vi "CountersVisualization.vi"(0 "Counters Monitor Array IN":T1(array[cluster]), 1 "SenderMail":string, 3 "ConnectionDSN":string, 4 "Password":string, 5 "Recipients":string, 6 "ArrayAlarmIN":bool[](array[boolean]), 7 "LineName":string, 9 "PLC Connection Array":T3(array[cluster]) {"PLC Type" items=["Keyence", "Allen Bradley", "Mitsubishi", "Panasonic", "Siemens"]}, 11 "OnlineStations":T2(array[cluster]), 13 "EmailsEnabled":string) -> (14 "Counters Monitor Array OUT":T1(array[cluster]), 19 "ArrayAlarmOUT":bool[](array[boolean]))   [LabVIEW 2017]
panel:
  in  "Tab Control":enum32{"Parameters", "Components", "Machines"}(tab)
  # "Online Monitor"
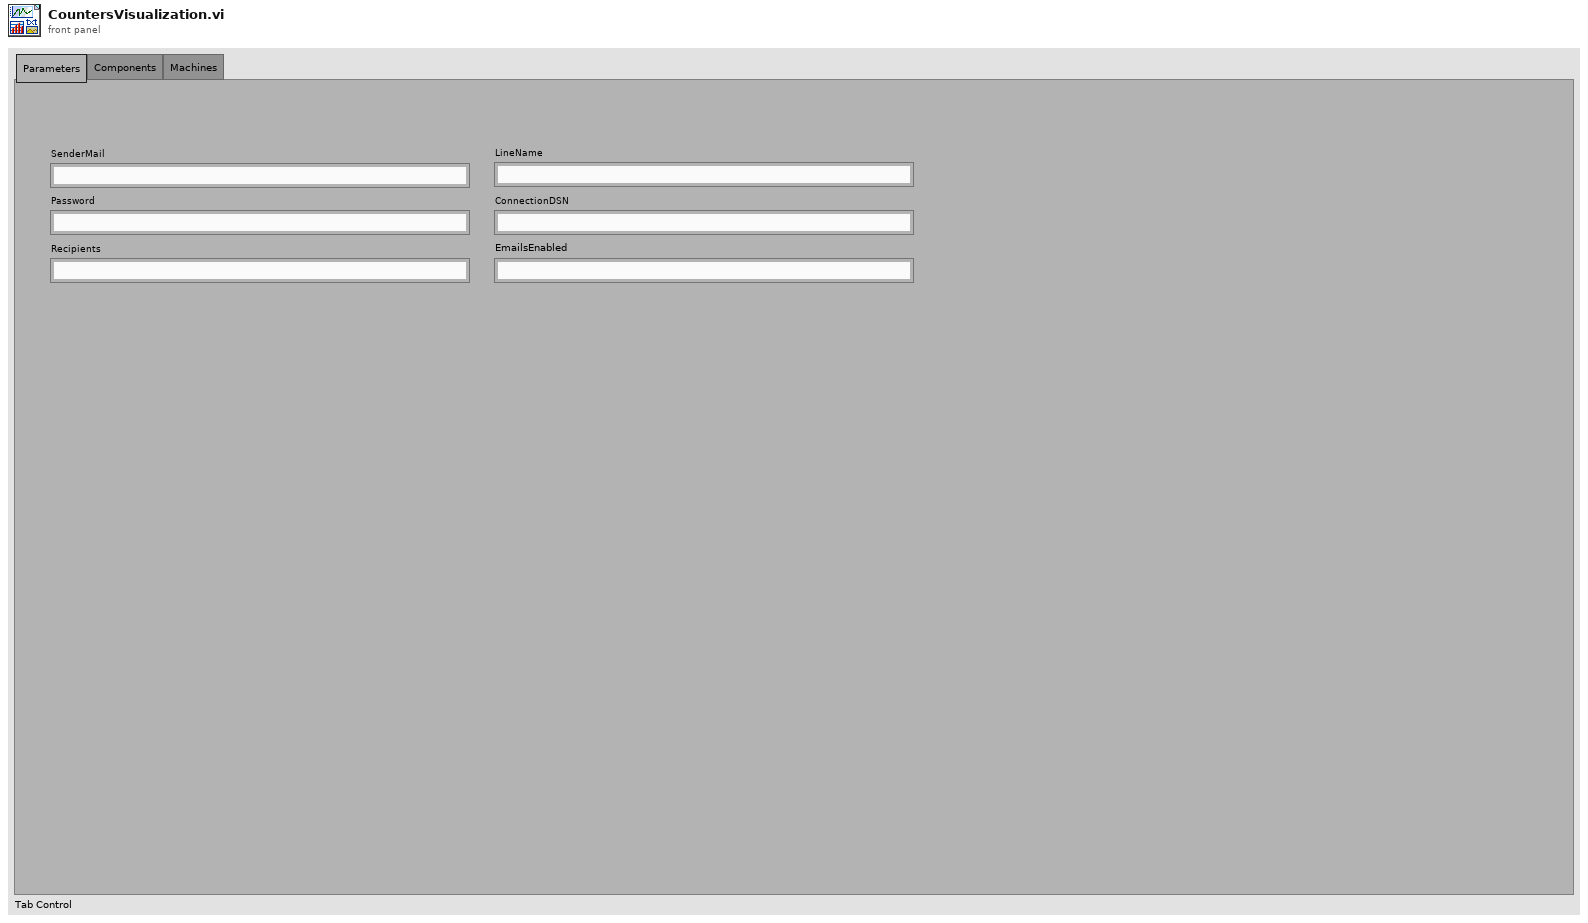
[diagram p1: front panel]
types:
  T1 = cluster{"MachineName":string, "ComponentName":string, "StoppageAlarmCounter":i32, "CurrentCount":i32, "StatusColorBox":u32, "ToolCribPartNumber":string}[]
  T2 = cluster{"Connection":bool, "MachineName":string}[]
  T3 = cluster{"MachineName":string, "PLC Address":string, "PLC Type":u16, "MemoryNumber1":string, "MemoryNumber2":string, "MemoryNumber3":string}[]
  T4 = enum8{"Enabled", "Disabled", "Disabled and Grayed Out"}
  T5 = cluster{"MachineName":string, "ComponentName":string, "StoppageAlarmCounter":i32, "CurrentCount":i32, "StatusColorBox":u32, "ToolCribPartNumber":string}
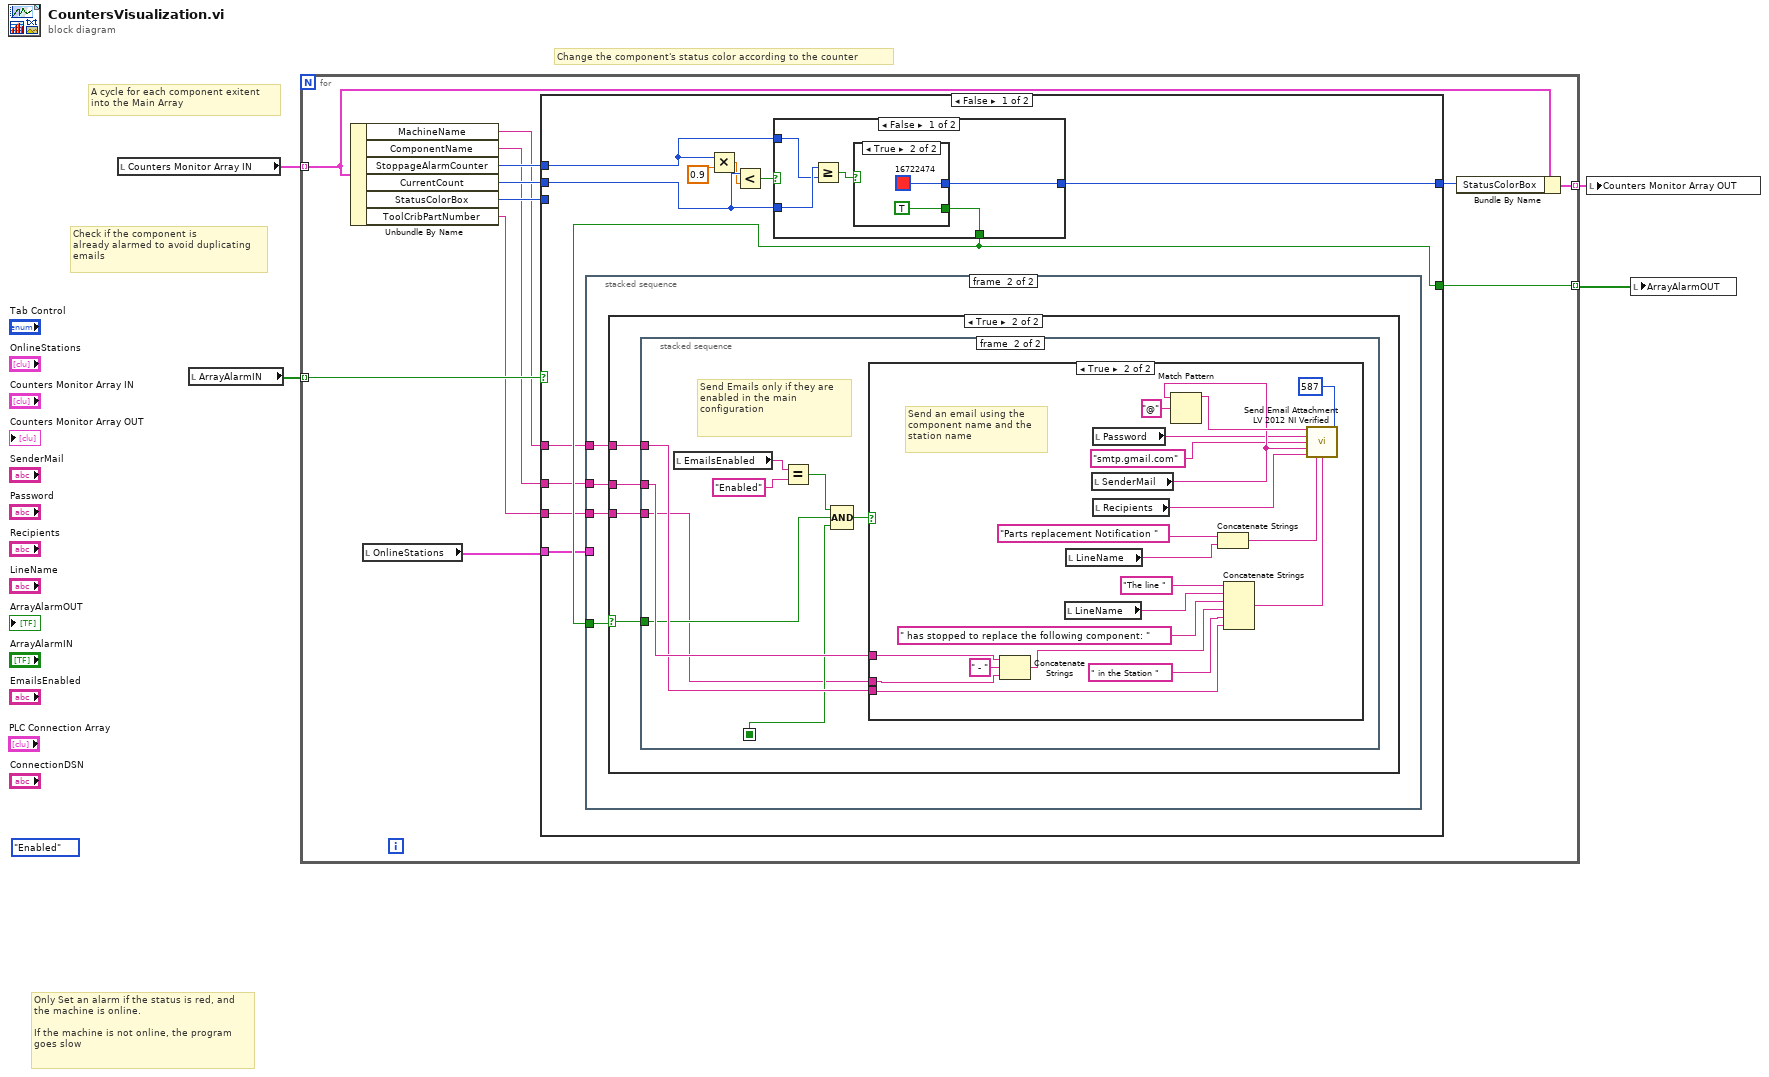
[diagram p0: block diagram]
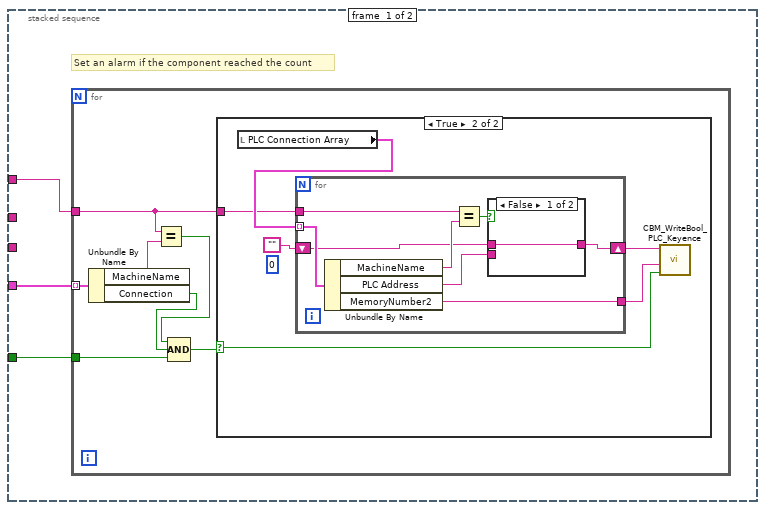
[diagram p2: hidden frame]
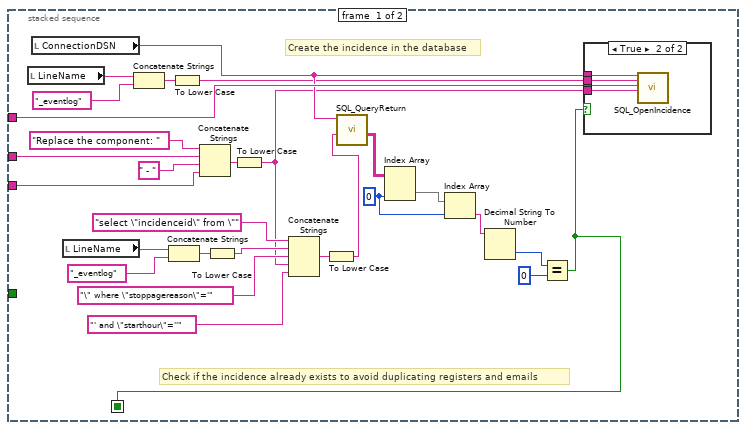
[diagram p6: hidden frame]
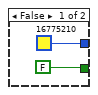
[diagram p9: hidden frame]
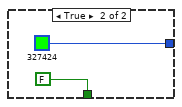
[diagram p10: hidden frame]
diagram:
  (unwired) T4."Enabled" ("Disabled")
  # "Only Set an alarm if the status is red, and\nthe machine is online.\n\nIf the machine is not online, the program \ngoes slow"
  # "Change the component's status color according to the counter"
  # "Check if the component is \nalready alarmed to avoid duplicating\nemails"
  # "A cycle for each component exitent\ninto the Main Array"
  n1 = local read "Counters Monitor Array IN"() -> (w4:T1)
  n2 = local read "ArrayAlarmIN"() -> (w2:bool[])
  n3 = for {
    tunnel: w4 -> [w16] mode=indexing
    tunnel: [w14] -> w3 mode=indexing
    tunnel: w2 -> [w12] mode=indexing
    tunnel: [w11] -> w1 mode=indexing
    n4 = Unbundle By Name(w16) -> ("MachineName"=w8:string, "ComponentName"=w6:string, "StoppageAlarmCounter"=w13:i32, "CurrentCount"=w10:i32, "StatusColorBox"=w9:u32, "ToolCribPartNumber"=w5:string)
    n5 = local read "OnlineStations"() -> (w7:T2)
    n6 = case shown="False" w12 {
      selector: w12 -> [_ w135]
      tunnel: [w25 w134] -> w15
      tunnel: w10 -> [w24 _]
      tunnel: w13 -> [w22 _]
      tunnel: [w21 w135] -> w11
      tunnel: w9 -> [_ w134]
      tunnel: w8 -> [w20 _]
      tunnel: w7 -> [w19 _]
      tunnel: w6 -> [w18 _]
      tunnel: w5 -> [w17 _]
      frame False {
        n7 = Multiply(x=w22, y=0.9) -> (x*y=w23:dbl)
        n8 = Less?(x=w24, y=w23) -> (x < y?=w26:bool)
        n9 = case shown="False" w26 {
          tunnel: [w124 u32 327424] -> w25
          tunnel: w24 -> [w127 _]
          tunnel: w22 -> [w126 _]
          tunnel: [w123 FALSE] -> w21
          frame False {
            n10 = Greater Or Equal?(x=w127, y=w126) -> (x >= y?=w125:bool)
            n11 = case shown="True" w125 {
              tunnel: [u32 16775210 u32 16722474] -> w124
              tunnel: [FALSE TRUE] -> w123
              frame False {
              }
              frame True {
              }
            }
          }
          frame True {
          }
        }
        n12 = stacked-sequence {
          tunnel: w21 -> [w30 w54]
          tunnel: w20 -> [w29 w57]
          tunnel: w19 -> [w28 _]
          tunnel: w18 -> [_ w56]
          tunnel: w17 -> [_ w55]
          frame #0 {
            # "Set an alarm if the component reached the count"
            n13 = for {
              tunnel: w30 -> [w31]
              tunnel: w29 -> [w36]
              tunnel: w28 -> [w37] mode=indexing
              n14 = Unbundle By Name(w37) -> ("MachineName"=w35:string, "Connection"=w32:bool)
              n15 = Equal?(x=w36, y=w35) -> (x = y?=w33:bool)
              n16 = Compound Arithmetic op=AND(w33, w32, w31) -> (w34:bool)
              n17 = case shown="True" w34 {
                selector: w34 -> [_ w41]
                tunnel: w36 -> [_ w42]
                frame False {
                }
                frame True {
                  (unwired) 0
                  n18 = local read "PLC Connection Array"() -> (w43:T3)
                  n19 = for {
                    tunnel: w43 -> [w51] mode=indexing
                    tunnel: w42 -> [w49]
                    shift-right: [w46] -> w40
                    shift-left: "" -> [w45]
                    tunnel: [w44] -> w38
                    n20 = Unbundle By Name(w51) -> ("MachineName"=w50:string, "PLC Address"=w47:string, "MemoryNumber2"=w44:string)
                    n21 = Equal?(x=w49, y=w50) -> (x = y?=w48:bool)
                    n22 = case shown="False" w48 {
                      tunnel: w47 -> [_ w53]
                      tunnel: [w52 w53] -> w46
                      tunnel: w45 -> [w52 _]
                      frame False {
                      }
                      frame True {
                      }
                    }
                  }
                  n23 = call "CBM_WriteBool_PLC_Keyence.vi"("Set?"=w41, "MemoryNumber"=w38, "PLC_IP"=w40) -> ()  [unwired: 8 in, 1 out]
                }
              }
            }
          }
          frame #1 {
            n24 = case shown="True" w54 {
              selector: w54 -> [_ w58]
              tunnel: w57 -> [_ w61]
              tunnel: w56 -> [_ w60]
              tunnel: w55 -> [_ w59]
              frame False {
              }
              frame True {
                n25 = stacked-sequence {
                  seq-local: [w62 _] -> [_ w96]
                  tunnel: w61 -> [w87 w101]
                  tunnel: w60 -> [w85 w102]
                  tunnel: w59 -> [w83 w94]
                  tunnel: w58 -> [_ w97]
                  frame #0 {
                    w70 = 0 ("disabled index (col)")
                    # "Check if the incidence already exists to avoid duplicating registers and emails"
                    # "Create the incidence in the database"
                    n26 = local read "LineName"() -> (w89:string)
                    n27 = local read "ConnectionDSN"() -> (w81:string)
                    n28 = local read "LineName"() -> (w76:string)
                    n29 = Concatenate Strings(w89, "_eventlog") -> (w82:string)
                    n30 = Concatenate Strings(w76, "_eventlog") -> (w78:string)
                    n31 = To Lower Case(string=w82) -> (all lower case string=w80:string)
                    n32 = Concatenate Strings("Replace the component: " ("Subject:"), w85, " - " ("Subject:"), w83) -> (w64:string)
                    n33 = To Lower Case(string=w78) -> (all lower case string=w75:string)
                    n34 = To Lower Case(string=w64) -> (all lower case string=w63:string)
                    n35 = Concatenate Strings("select \"incidenceid\" from \"", w75, "\" where \"stoppagereason\"='", w63, "' and \"starthour\"=''") -> (w69:string)
                    n36 = To Lower Case(string=w69) -> (all lower case string=w68:string)
                    n37 = call "SQL_QueryReturn.vi"("SQL query"=w68, "ConnectionDSN"=w81) -> ("data"=w72:string[][])  [unwired: 9 in]
                    n38 = Index Array(array=w72, index (col)=w70) -> (element=w71:string[])  [unwired: 1 in]
                    n39 = Index Array(array=w71, index=w70) -> (element=w67:string)
                    n40 = Decimal String To Number(string=w67) -> (number=w66:i32)  [unwired: 2 in, 1 out]
                    n41 = Equal?(x=w66, y=0) -> (x = y?=w62:bool)
                    n42 = case shown="True" w62 {
                      tunnel: w81 -> [_ w93]
                      tunnel: w87 -> [_ w92]
                      tunnel: w63 -> [_ w91]
                      tunnel: w80 -> [_ w90]
                      frame False {
                      }
                      frame True {
                        n43 = call "SQL_OpenIncidence.vi"("ConnectionDSN"=w93, "TableName"=w90, "MachineName"=w92, "StoppageReason"=w91) -> ()  [unwired: 16 in]
                      }
                    }
                  }
                  frame #1 {
                    # "Send Emails only if they are enabled in the main\nconfiguration"
                    n44 = local read "EmailsEnabled"() -> (w100:string)
                    n45 = Equal?(x=w100, y="Enabled") -> (x = y?=w98:bool)
                    n46 = Compound Arithmetic op=AND(w98, w97, w96) -> (w95:bool)
                    n47 = case shown="True" w95 {
                      tunnel: w102 -> [_ w106]
                      tunnel: w101 -> [_ w108]
                      tunnel: w94 -> [_ w104]
                      frame False {
                      }
                      frame True {
                        # "Send an email using the \ncomponent name and the\nstation name"
                        n48 = Concatenate Strings(w106, " - " ("string"), w104) -> (w103:string)
                        n49 = local read "LineName"() -> (w111:string)
                        n50 = local read "LineName"() -> (w114:string)
                        n51 = local read "SenderMail"() -> (w119:string)
                        n52 = local read "Password"() -> (w118:string)
                        n53 = local read "Recipients"() -> (w116:string)
                        n54 = Match Pattern(string=w119, regular expression="@") -> (before substring=w120:string)  [unwired: 1 in, 3 out]
                        n55 = Concatenate Strings("Parts replacement Notification " ("Subject:"), w114) -> (w113:string)
                        n56 = Concatenate Strings("The line " ("Subject:"), w111, " has stopped to replace the following component: " ("Subject:"), w103, " in the Station " ("Subject:"), w108) -> (w107:string)
                        n57 = call "Send Email Attachment LV 2012 NI Verified.vi"("Email Account ID"=w120, "Port"=587, "Email Account Password"=w118, "SMTP Outgoing Mail Server"="smtp.gmail.com", "From: (email@site.com)"=w119, "To: (email@site.com)"=w116, "Subject:"=w113, "Body:"=w107) -> ()  [unwired: 7 in, 1 out]
                      }
                    }
                  }
                }
              }
            }
          }
        }
      }
      frame True {
      }
    }
    n58 = Bundle By Name(cluster=w16, "StatusColorBox"=w15) -> (w14:T5)
  }
  n59 = local write "Counters Monitor Array OUT"(w3) -> ()
  n60 = local write "ArrayAlarmOUT"(w1) -> ()
